vi "Add_Signal.vi"(10 "CAN_MSGs":T1={"Scaling Factor"=1, "Physical value"=0.0, "CAN_Frames"={"CAN_ID"=0, "MSGTYPE"=128, "Payload"=[], "Length"=0}, "Offset value"=0.0, "Framing datas"=[], "CAN_Frame Enable"=FALSE, "Add Signal"=FALSE, "Delete Signal"=FALSE, "Signal Values"=[], "Time(ms)"=0.0, "Repetition"=FALSE, "Delay"=FALSE, "Delay time"=0.0} {"CAN_Frames"."Payload" format="%.0x"; "CAN_Frames"."MSGTYPE" items=["STATUS"=128, "EXTENDED"=2, "RTR"=1, "DATA MSG"=0]; "CAN_Frames"."CAN_ID" format="%.0x"}) -> (2 "CAN_MSGs 2":T1={"Scaling Factor"=1, "Physical value"=0.0, "CAN_Frames"={"CAN_ID"=0, "MSGTYPE"=128, "Payload"=[], "Length"=0}, "Offset value"=0.0, "Framing datas"=[], "CAN_Frame Enable"=FALSE, "Add Signal"=FALSE, "Delete Signal"=FALSE, "Signal Values"=[], "Time(ms)"=0.0, "Repetition"=FALSE, "Delay"=FALSE, "Delay time"=0.0} {"CAN_Frames"."Payload" format="%.0x"; "CAN_Frames"."MSGTYPE" items=["STATUS"=128, "EXTENDED"=2, "RTR"=1, "DATA MSG"=0]; "CAN_Frames"."CAN_ID" format="%.0x"})   [LabVIEW 2024, in "PCANusb_DTU.lvlib"]
uses:
  PCANusb_DTU.lvlib
  CAN_MSGs.ctl
  CAN_Frames_ctrl.ctl
  Framing datas.ctl
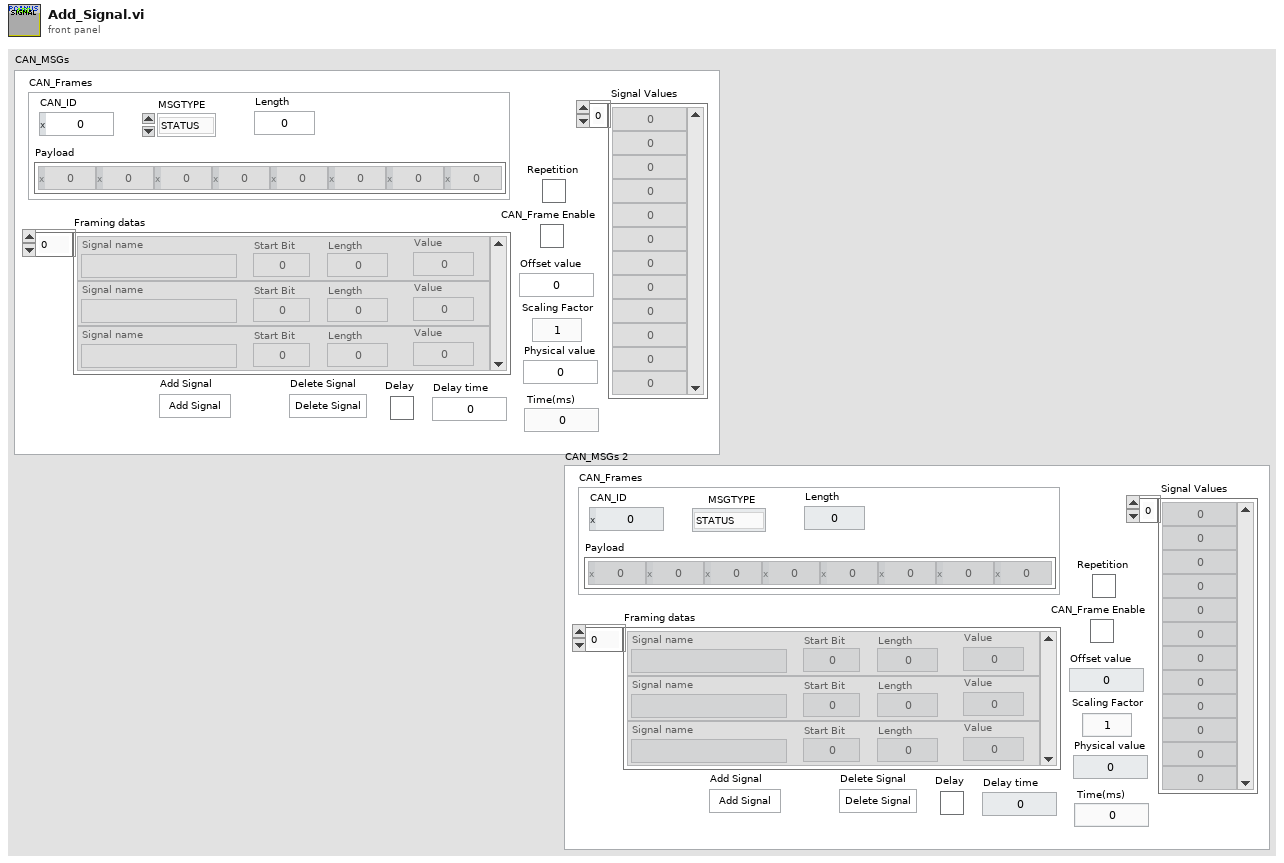
[diagram p1: front panel]
types:
  T1 = typedef "PCANusb_DTU.lvlib/CAN_MSGs.ctl" = cluster{"Scaling Factor":u16, "Physical value":dbl, "CAN_Frames":T2, "Offset value":dbl, "Framing datas":T3[], "CAN_Frame Enable":bool, "Add Signal":bool, "Delete Signal":bool, "Signal Values":dbl[], "Time(ms)":dbl, "Repetition":bool, "Delay":bool, "Delay time":dbl}
  T2 = typedef "PCANusb_DTU.lvlib/CAN_Frames_ctrl.ctl" = cluster{"CAN_ID":u32, "MSGTYPE":u8, "Payload":u8[], "Length":u8}
  T3 = typedef "PCANusb_DTU.lvlib/Framing datas.ctl" = cluster{"Signal name":string, "Start Bit":u8, "Length":u8, "Value":u16}
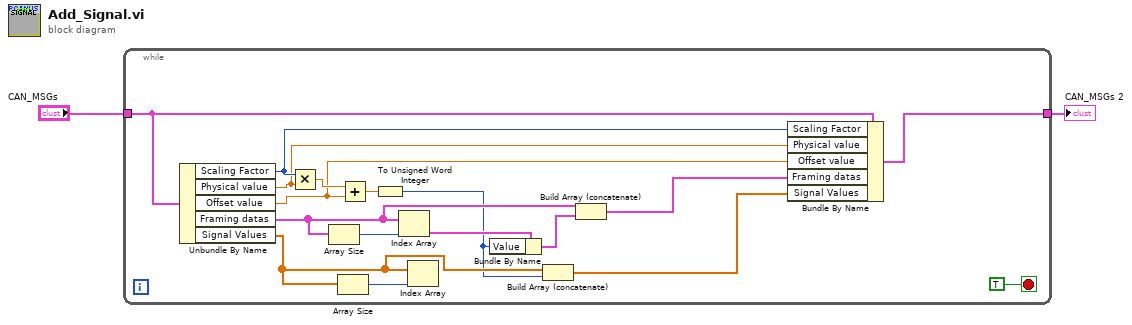
[diagram p0: block diagram]
diagram:
  n1 = while {
    tunnel: "CAN_MSGs" -> [w18]
    tunnel: [w15] -> w1
    stop <- TRUE stop-if-true
    n2 = Unbundle By Name(w18) -> ("Scaling Factor"=w14:u16, "Physical value"=w13:dbl, "Offset value"=w12:dbl, "Framing datas"=w10:T3[], "Signal Values"=w5:dbl[])
    n3 = Multiply(x=w14, y=w13) -> (x*y=w17:dbl)
    n4 = Array Size(array=w10) -> (size(s)=w11:i32)
    n5 = Array Size(array=w5) -> (size(s)=w7:i32)
    n6 = Add(x=w17, y=w12) -> (x+y=w16:dbl)
    n7 = To Unsigned Word Integer(number=w16) -> (unsigned 16bit integer=w3:u16)
    n8 = Index Array(array=w10, index=w11) -> (element=w8:T3)
    n9 = Index Array(array=w5, index=w7) -> ()  [unwired: 1 out]
    n10 = Bundle By Name(cluster=w8, "Value"=w3) -> (w6:T3)
    n11 = Build Array (concatenate)(w5, w3) -> (w4:dbl[])
    n12 = Build Array (concatenate)(w10, w6) -> (w9:T3[])
    n13 = Bundle By Name(cluster=w18, "Scaling Factor"=w14, "Physical value"=w13, "Offset value"=w12, "Framing datas"=w9, "Signal Values"=w4) -> (w15:T1)
  }
  "CAN_MSGs 2" <- w1
